vi "Frequency.vi"(11 "New Value":bool) -> (3 "RPM":sgl)   [LabVIEW 2018]
panel:
  out "Frequency(Hz)":sgl
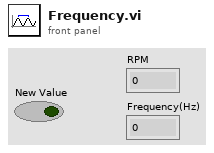
[diagram p1: front panel]
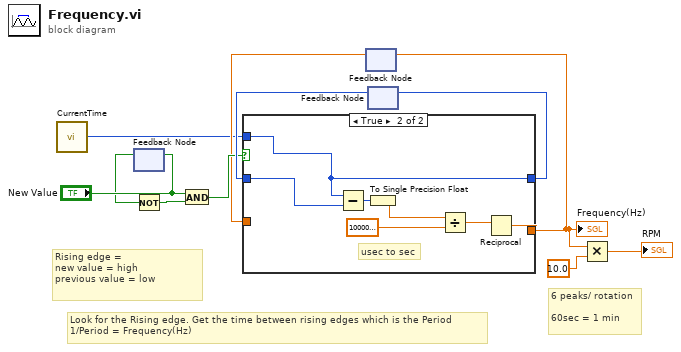
[diagram p0: block diagram]
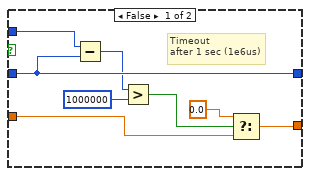
[diagram p2: hidden frame]
diagram:
  # "6 peaks/ rotation\n\n60sec = 1 min"
  # "Look for the Rising edge. Get the time between rising edges which is the Period\n1/Period = Frequency(Hz)"
  # "Rising edge =\nnew value = high\nprevious value = low"
  n1 = call "CurrentTime"() -> ("Tick Count(uSec)"=w3:u32)
  n2 = feedback #1() -> (w1:bool)  [unwired: 1 in]
  n3 = feedback-in #1("New Value") -> ()
  n4 = Not(x=w1) -> (.not. x?=w7:bool)
  n5 = And(x="New Value", y=w7) -> (x .and. y?=w9:bool)
  n6 = feedback #2() -> (w8:sgl)  [unwired: 1 in]
  n7 = feedback #3() -> (w11:u32)  [unwired: 1 in]
  n8 = case shown="True" w9 {
    tunnel: [w18 w20] -> w10
    tunnel: w11 -> [w18 w26]
    tunnel: [w14 w24] -> w6
    tunnel: w8 -> [w13 _]
    tunnel: w3 -> [w19 w20]
    frame False {
      # "Timeout\nafter 1 sec (1e6us)"
      n9 = Subtract(x=w19, y=w18) -> (x-y=w17:u32)
      n10 = Greater?(x=w17, y=u32 1000000) -> (0:w15:bool)
      n11 = Select(t=sgl 0.0, s=w15, f=w13) -> (s? t:f=w14:sgl)
    }
    frame True {
      # "usec to sec"
      n12 = Subtract(x=w20, y=w26) -> (x-y=w22:u32)
      n13 = To Single Precision Float(number=w22) -> (single precision float=w21:sgl)
      n14 = Divide(x=w21, y=sgl 1000000.0) -> (x/y=w23:sgl)
      n15 = Reciprocal(x=w23) -> (1/x=w24:sgl)
    }
  }
  "Frequency(Hz)" <- w6
  n16 = feedback-in #2(w6) -> ()
  n17 = feedback-in #3(w10) -> ()
  n18 = Multiply(x=w6, y=sgl 10.0) -> (x*y=→"RPM":sgl)
